vi "Set Error Message.vi"(4 "enable (T)":bool=TRUE, 5 "error in":errorcluster, 6 "append time (F)":bool, 7 "code (-1)":i32=-1, 8 "message":string="User error message.") -> (0 "error out":errorcluster {"code" format="%.0x"})   [LabVIEW 2020]
doc: "If enabled (default), set the error status, code, and message values."
panel:
  # "(trim period, append \" at \", current time AM/PM, period\nExample \"at 10:21 AM.\")"
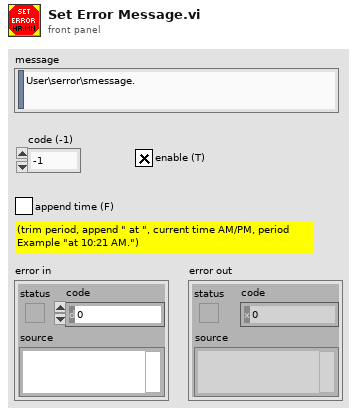
[diagram p1: front panel]
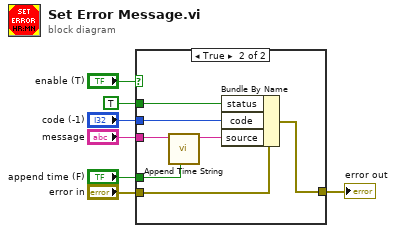
[diagram p0: block diagram]
diagram:
  n1 = case shown="True" "enable (T)" {
    tunnel: "code (-1)" -> [_ w15]
    tunnel: TRUE ("status") -> [_ w14]
    tunnel: [w8 w9] -> w5
    tunnel: "error in" -> [w8 w10]
    tunnel: "append time (F)" -> [_ w11]
    tunnel: "message" -> [_ w12]
    frame False {
    }
    frame True {
      n2 = call "Append Time String.vi"("enable (T)"=w11, "string in"=w12) -> ("string out"=w13:string)  [unwired: 5 in, 1 out]
      n3 = Bundle By Name(cluster=w10, "status"=w14, "code"=w15, "source"=w13) -> (w9:errorcluster)
    }
  }
  "error out" <- w5
